vi "Correlation.vi"(6 "zero lag +":i32=1, 7 "Time step (ms)":dbl, 9 "AC final pts":i32, 10 "counts/bin":dbl[](array[numeric]), 11 "mean":dbl) -> (0 "Time":dbl[](array[numeric]), 3 "Data out":dbl[](array[numeric]))   [LabVIEW 2022 SP3]
uses:
  <vilib>/Analysis/2dsp.llb/1D Cross Correlation (DBL).vi
  <vilib>/Analysis/NI_AALPro.lvlib
panel:
  out "Data out 2":dbl[](array[numeric])
  out "elements":dbl[](array[numeric])
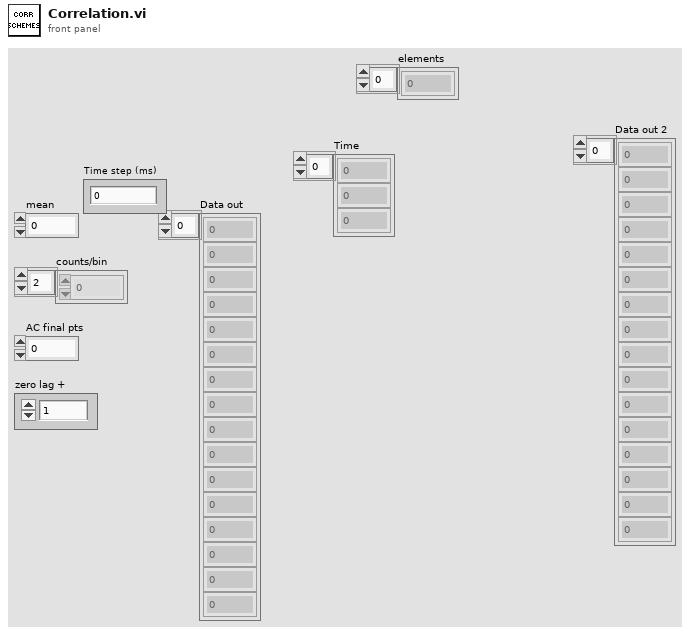
[diagram p1: front panel]
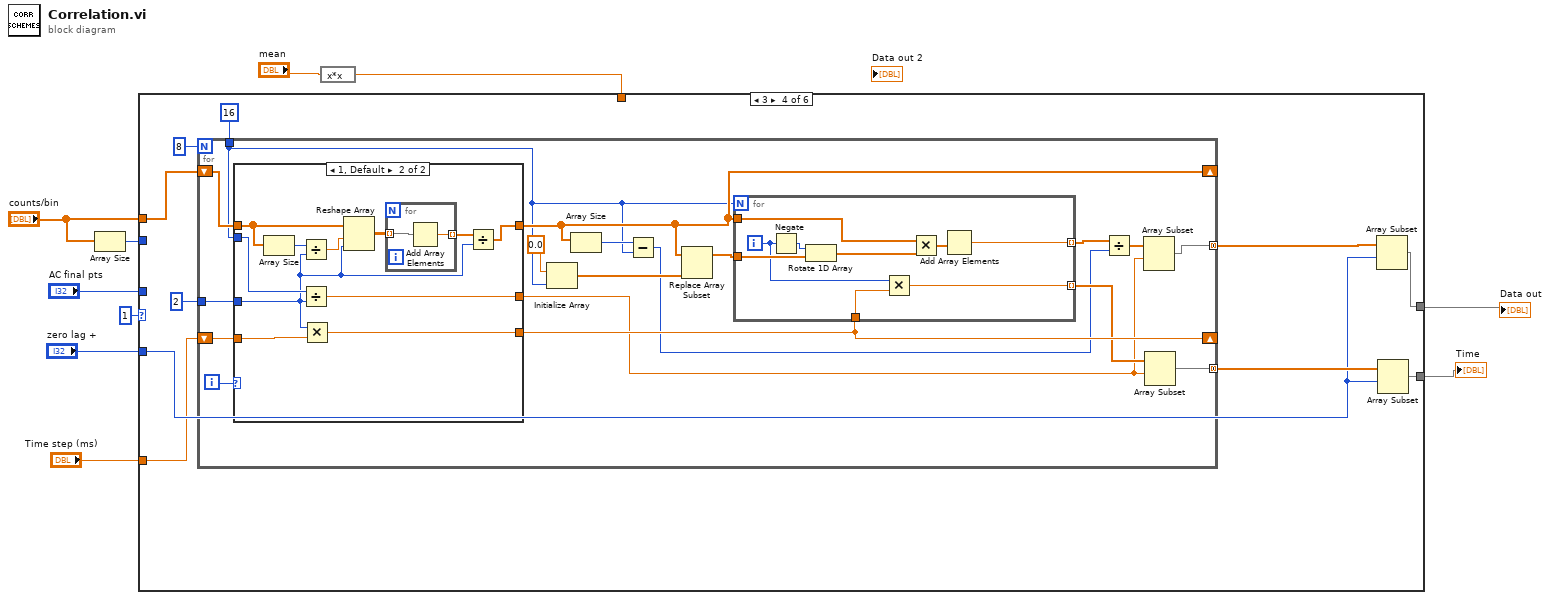
[diagram p0: block diagram]
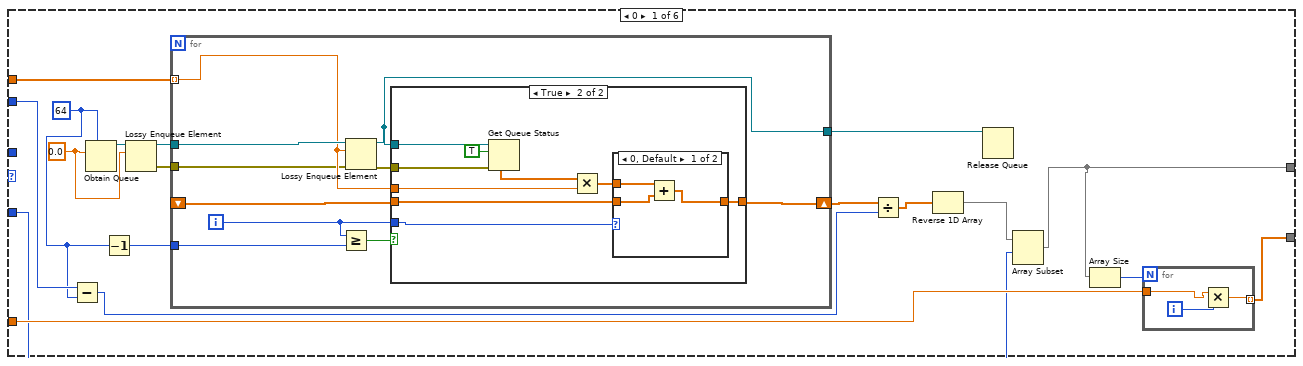
[diagram p2: hidden frame]
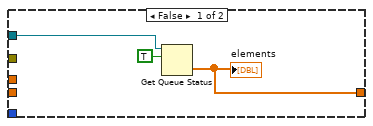
[diagram p3: hidden frame]
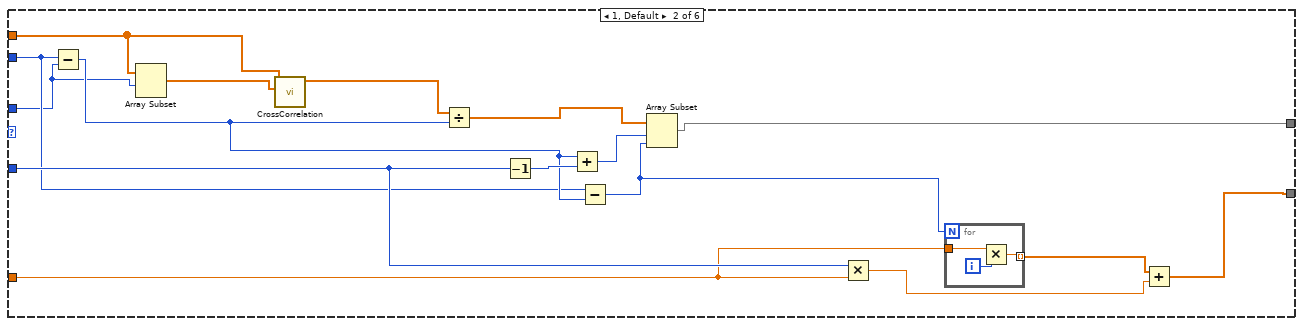
[diagram p5: hidden frame]
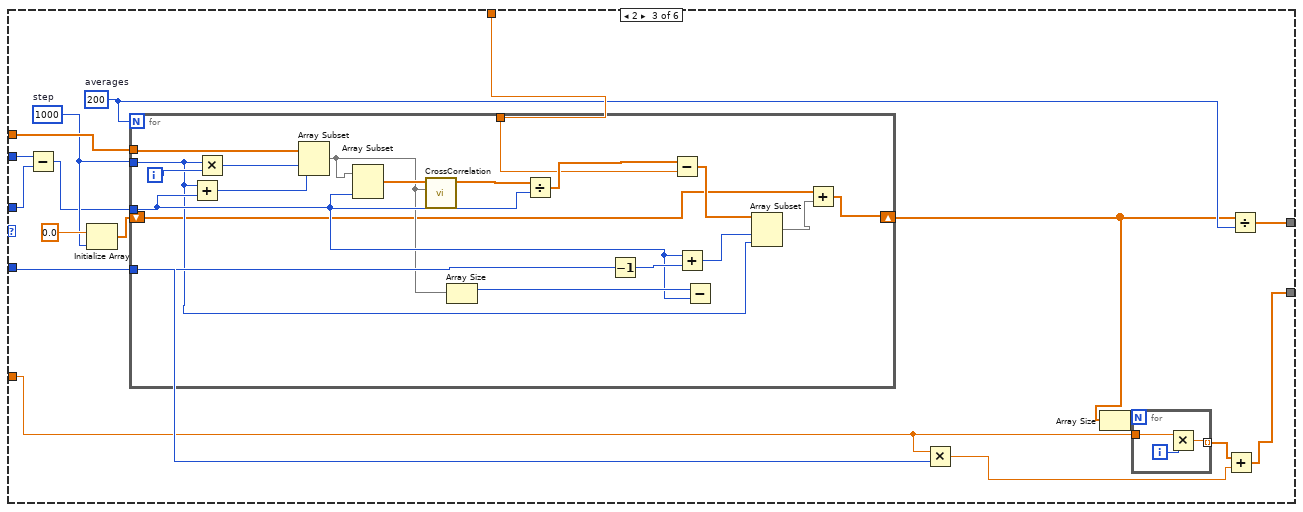
[diagram p6: hidden frame]
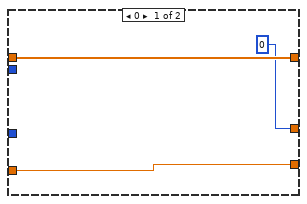
[diagram p7: hidden frame]
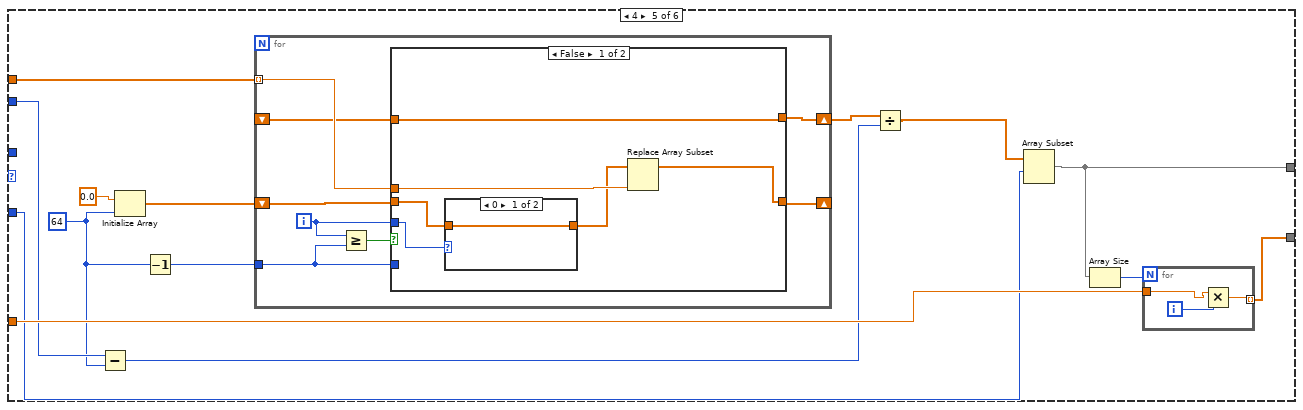
[diagram p8: hidden frame]
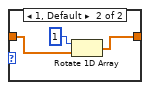
[diagram p9: hidden frame]
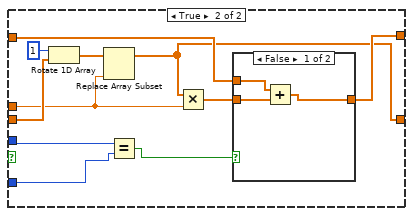
[diagram p10: hidden frame]
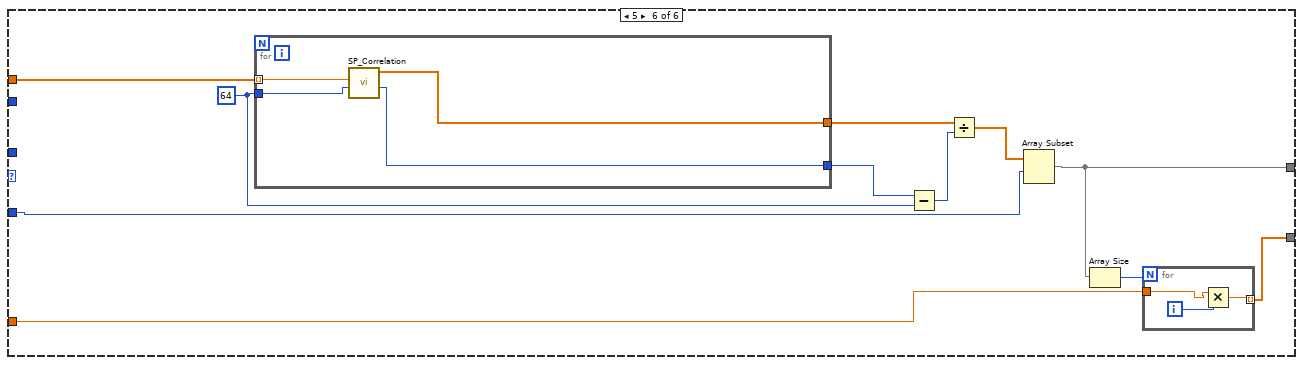
[diagram p12: hidden frame]
diagram:
  n1 = Array Size(array="counts/bin") -> (size(s)=w1:i32)
  n2 = expression code="x*x"("mean") -> (w5:dbl)
  n3 = case shown="3" 1 {
    tunnel: [w17 w58 w90 w121 w170 w223] -> w10
    tunnel: w5 -> [_ _ w93 _ _ _]
    tunnel: "AC final pts" -> [_ w62 w77 _ _ _]
    tunnel: "counts/bin" -> [w28 w60 w92 w125 w182 w229]
    tunnel: "zero lag +" -> [w15 w67 w85 w119 w171 w224]
    tunnel: "Time step (ms)" -> [w25 w66 w84 w118 w180 w227]
    tunnel: [w24 w65 w81 w117 w179 w226] -> w3
    tunnel: w1 -> [w22 w63 w79 _ w175 _]
    frame 0 {
      w11 = 0.0 ("mean")
      w16 = 64 ("max queue size (-1, unlimited)")
      n4 = Subtract(x=w22, y=w16) -> (x-y=w19:i32)
      n5 = Obtain Queue(max queue size (-1, unlimited)=w16, element data type=w11) -> (queue out=w14:refnum<queue>)  [unwired: 3 in, 2 out]
      n6 = Decrement(x=w16) -> (x-1=w23:i32)
      n7 = Lossy Enqueue Element(queue=w14, element=w11) -> (queue out=w13:refnum<queue>, error out=w12:errorcluster)  [unwired: 1 in, 2 out]
      n8 = for {
        tunnel: w28 -> [w37] mode=indexing
        tunnel: w13 -> [w41]
        shift-right: [w39] -> w21
        shift-left: _ -> [w40]
        tunnel: w23 -> [w38]
        tunnel: [w36] -> w27
        tunnel: w12 -> [w32]
        i -> [w33]
        n9 = Greater Or Equal?(x=w33, y=w38) -> (x >= y?=w34:bool)
        n10 = Lossy Enqueue Element(queue=w41, element=w37, error in (no error)=w32) -> (queue out=w36:refnum<queue>, error out=w35:errorcluster)  [unwired: 2 out]
        n11 = case shown="True" w34 {
          tunnel: w36 -> [w43 w53]
          tunnel: w37 -> [_ w45]
          tunnel: w40 -> [_ w52]
          tunnel: [w42 w51] -> w39
          tunnel: w35 -> [_ w50]
          tunnel: w33 -> [_ w47]
          frame False {
            n12 = Get Queue Status(queue=w43, return elements? (F)=TRUE) -> (elements=w42:dbl[])  [unwired: 1 in, 7 out]
            "elements" <- w42
          }
          frame True {
            n13 = Get Queue Status(queue=w53, return elements? (F)=TRUE, error in (no error)=w50) -> (elements=w46:dbl[])  [unwired: 7 out]
            n14 = Multiply(x=w46, y=w45) -> (x*y=w48:dbl[])
            n15 = case shown="0, Default" w47 {
              tunnel: w52 -> [w56 _]
              tunnel: [w54 w57] -> w51
              tunnel: w48 -> [w55 w57]
              frame 0, Default {
                n16 = Add(x=w55, y=w56) -> (x+y=w54:dbl[])
              }
              frame 16 {
              }
            }
          }
        }
      }
      n17 = Divide(x=w21, y=w19) -> (x/y=w20:dbl[])
      n18 = Reverse 1D Array(array=w20) -> (reversed array=w18:dbl[])
      n19 = Release Queue(queue=w27) -> ()  [unwired: 2 in, 3 out]
      n20 = Array Subset(array=w18, index=w15) -> (w17:dbl[])  [unwired: 1 in]
      n21 = Array Size(array=w17) -> (size(s)=w26:i32)
      n22 = for {
        N: w26 -> [_]
        tunnel: [w30] -> w24 mode=indexing
        tunnel: w25 -> [w29]
        i -> [w31]
        n23 = Multiply(x=w29, y=w31) -> (x*y=w30:dbl)
      }
    }
    frame 1, Default {
      n24 = Subtract(x=w63, y=w62) -> (x-y=w64:i32)
      n25 = Array Subset(array=w60, index=w62) -> (w61:dbl[])  [unwired: 1 in]
      n26 = call-poly <vilib>:"CrossCorrelation.vi"("Y"=w61, "X"=w60) -> ("Rxy"=w71:dbl[])  [unwired: 8 in, 1 out]
      n27 = Divide(x=w71, y=w64) -> (x/y=w59:dbl[])
      n28 = Decrement(x=w67) -> (x-1=w73:i32)
      n29 = Add(x=w64, y=w73) -> (x+y=w72:i32)
      n30 = Subtract(x=w63, y=w64) -> (x-y=w68:i32)
      n31 = Array Subset(array=w59, index=w72, length=w68) -> (w58:dbl[])
      n32 = Multiply(x=w67, y=w66) -> (x*y=w70:dbl)
      n33 = for {
        N: w68 -> [_]
        tunnel: [w75] -> w69 mode=indexing
        tunnel: w66 -> [w74]
        i -> [w76]
        n34 = Multiply(x=w74, y=w76) -> (x*y=w75:dbl)
      }
      n35 = Add(x=w69, y=w70) -> (x+y=w65:dbl[])
    }
    frame 2 {
      w80 = 1000  # step
      w91 = 200  # averages
      n36 = Subtract(x=w79, y=w77) -> (x-y=w78:i32)
      n37 = Initialize Array(0.0 ("mean"), w80) -> (w89:dbl[])
      n38 = for {
        N: w91 -> [_]
        tunnel: w78 -> [w103]
        tunnel: w85 -> [w110]
        tunnel: w93 -> [w107]
        tunnel: w92 -> [w106]
        tunnel: w80 -> [w100]
        shift-right: [w98] -> w86
        shift-left: w89 -> [w97]
        i -> [w105]
        n39 = Add(x=w100, y=w103) -> (x+y=w102:i32)
        n40 = Multiply(x=w100, y=w105) -> (x*y=w104:i32)
        n41 = Array Subset(array=w106, index=w104, length=w102) -> (w101:dbl[])
        n42 = Array Subset(array=w101, length=w103) -> (w113:dbl[])  [unwired: 1 in]
        n43 = call-poly <vilib>:"CrossCorrelation.vi"("Y"=w101, "X"=w113) -> ("Rxy"=w112:dbl[])  [unwired: 8 in, 1 out]
        n44 = Array Size(array=w101) -> (size(s)=w111:i32)
        n45 = Divide(x=w112, y=w103) -> (x/y=w109:dbl[])
        n46 = Decrement(x=w110) -> (x-1=w115:i32)
        n47 = Subtract(x=w109, y=w107) -> (x-y=w108:dbl[])
        n48 = Add(x=w103, y=w115) -> (x+y=w114:i32)
        n49 = Subtract(x=w111, y=w103) -> ()  [unwired: 1 out]
        n50 = Array Subset(array=w108, index=w114, length=w100) -> (w99:dbl[])
        n51 = Add(x=w97, y=w99) -> (x+y=w98:dbl[])
      }
      n52 = Multiply(x=w84, y=w85) -> (x*y=w83:dbl)
      n53 = Array Size(array=w86) -> (size(s)=w87:i32)
      n54 = for {
        N: w87 -> [_]
        tunnel: [w95] -> w82 mode=indexing
        tunnel: w84 -> [w94]
        i -> [w96]
        n55 = Multiply(x=w94, y=w96) -> (x*y=w95:dbl)
      }
      n56 = Add(x=w82, y=w83) -> (x+y=w81:dbl[])
      n57 = Divide(x=w86, y=w91) -> (x/y=w90:dbl[])
    }
    frame 3 {
      n58 = for {
        N: 8 -> [_]
        shift-right: [w138] -> _
        shift-left: w125 -> [w139]
        tunnel: 2 -> [w135]
        tunnel: [w128] -> w122 mode=concatenating
        shift-right: [w132] -> _
        shift-left: w118 -> [w133]
        tunnel: [w129] -> w120 mode=concatenating
        tunnel: 16 -> [w126]
        i -> [w134]
        n59 = case shown="1, Default" w134 {
          tunnel: w139 -> [w146 w153]
          tunnel: [w146 w147] -> w138
          tunnel: w135 -> [_ w149]
          tunnel: [0 w150] -> w130
          tunnel: w133 -> [w144 w154]
          tunnel: [w144 w152] -> w132
          tunnel: w126 -> [_ w151]
          frame 0 {
          }
          frame 1, Default {
            n60 = Array Size(array=w153) -> (size(s)=w157:i32)
            n61 = Divide(x=w157, y=w149) -> (x/y=w156:dbl)
            n62 = Divide(x=w151, y=w149) -> (x/y=w150:dbl)
            n63 = Multiply(x=w149, y=w154) -> (x*y=w152:dbl)
            n64 = Reshape Array(w153, w156, w149) -> (w155:dbl[][])
            n65 = for {
              tunnel: w155 -> [w159] mode=indexing
              tunnel: [w158] -> w148 mode=indexing
              n66 = Add Array Elements(numeric array=w159) -> (sum=w158:dbl)
            }
            n67 = Divide(x=w148, y=w149) -> (x/y=w147:dbl[])
          }
        }
        n68 = Initialize Array(0.0 ("mean"), w126) -> (w142:dbl[])
        n69 = Array Size(array=w138) -> (size(s)=w141:i32)
        n70 = Subtract(x=w141, y=w126) -> (x-y=w127:i32)
        n71 = Replace Array Subset(array=w138, new element=w142) -> (w140:dbl[])  [unwired: 1 in]
        n72 = for {
          N: w126 -> [_]
          tunnel: w138 -> [w165]
          tunnel: [w168] -> w137 mode=indexing
          tunnel: w140 -> [w164]
          tunnel: w132 -> [w163]
          tunnel: [w161] -> w131 mode=indexing
          i -> [w162]
          n73 = Negate(x=w162) -> (-x=w160:i32)
          n74 = Rotate 1D Array(1:w164, 2:w160) -> (0:w166:dbl[])
          n75 = Multiply(x=w162, y=w163) -> (x*y=w161:dbl)
          n76 = Multiply(x=w165, y=w166) -> (x*y=w167:dbl[])
          n77 = Add Array Elements(numeric array=w167) -> (sum=w168:dbl)
        }
        n78 = Divide(x=w137, y=w127) -> (x/y=w136:dbl[])
        n79 = Array Subset(array=w136, index=w130) -> (w128:dbl[])  [unwired: 1 in]
        n80 = Array Subset(array=w131, index=w130) -> (w129:dbl[])  [unwired: 1 in]
      }
      n81 = Array Subset(array=w122, index=w119) -> (w121:dbl[])  [unwired: 1 in]
      n82 = Array Subset(array=w120, index=w119) -> (w117:dbl[])  [unwired: 1 in]
    }
    frame 4 {
      w174 = 64 ("max queue size (-1, unlimited)")
      n83 = Subtract(x=w175, y=w174) -> (x-y=w173:i32)
      n84 = Initialize Array(0.0 ("dimension size"), w174) -> (w177:dbl[])
      n85 = Decrement(x=w174) -> (x-1=w176:i32)
      n86 = for {
        tunnel: w182 -> [w191] mode=indexing
        shift-right: [w192] -> _
        shift-left: w177 -> [w193]
        shift-right: [w189] -> w172
        shift-left: _ -> [w188]
        tunnel: w176 -> [w186]
        i -> [w187]
        n87 = Greater Or Equal?(x=w187, y=w186) -> (x >= y?=w190:bool)
        n88 = case shown="False" w190 {
          tunnel: w191 -> [w199 w207]
          tunnel: w193 -> [w197 w214]
          tunnel: [w195 w208] -> w192
          tunnel: [w194 w211] -> w189
          tunnel: w188 -> [w194 w210]
          tunnel: w187 -> [w198 w206]
          tunnel: w186 -> [_ w204]
          frame False {
            n89 = case shown="0" w198 {
              tunnel: w197 -> [w200 w202]
              tunnel: [w200 w201] -> w196
              frame 0 {
              }
              frame 1, Default {
                n90 = Rotate 1D Array(1:w202, 2:1 ("n")) -> (0:w201:dbl[])
              }
            }
            n91 = Replace Array Subset(array=w196, new element=w199) -> (w195:dbl[])  [unwired: 1 in]
          }
          frame True {
            n92 = Rotate 1D Array(1:w214, 2:1 ("n")) -> (0:w212:dbl[])
            n93 = Replace Array Subset(array=w212, new element=w207) -> (w208:dbl[])  [unwired: 1 in]
            n94 = Equal?(x=w206, y=w204) -> (x = y?=w205:bool)
            n95 = Multiply(x=w208, y=w207) -> (x*y=w213:dbl[])
            n96 = case shown="False" w205 {
              tunnel: w213 -> [w217 w218]
              tunnel: [w215 w218] -> w211
              tunnel: w210 -> [w216 _]
              frame False {
                n97 = Add(x=w216, y=w217) -> (x+y=w215:dbl[])
              }
              frame True {
              }
            }
          }
        }
      }
      n98 = Divide(x=w172, y=w173) -> (x/y=w169:dbl[])
      n99 = Array Subset(array=w169, index=w171) -> (w170:dbl[])  [unwired: 1 in]
      n100 = Array Size(array=w170) -> (size(s)=w181:i32)
      n101 = for {
        N: w181 -> [_]
        tunnel: [w184] -> w179 mode=indexing
        tunnel: w180 -> [w183]
        i -> [w185]
        n102 = Multiply(x=w183, y=w185) -> (x*y=w184:dbl)
      }
    }
    frame 5 {
      w221 = 64 ("max queue size (-1, unlimited)")
      n103 = for {
        tunnel: w229 -> [w236] mode=indexing
        tunnel: w221 -> [w235]
        tunnel: [w234] -> w220
        tunnel: [w233] -> w219
        n104 = call "SP_Correlation.vi"("Tau Number"=w235, "New Count"=w236) -> ("interation"=w233:i64, "Cross Corr"=w234:dbl[])  [unwired: 8 in]
      }
      n105 = Subtract(x=w219, y=w221) -> (x-y=w225:i64)
      n106 = Divide(x=w220, y=w225) -> (x/y=w222:dbl[])
      n107 = Array Subset(array=w222, index=w224) -> (w223:dbl[])  [unwired: 1 in]
      n108 = Array Size(array=w223) -> (size(s)=w228:i32)
      n109 = for {
        N: w228 -> [_]
        tunnel: [w231] -> w226 mode=indexing
        tunnel: w227 -> [w230]
        i -> [w232]
        n110 = Multiply(x=w230, y=w232) -> (x*y=w231:dbl)
      }
    }
  }
  "Data out" <- w10
  "Time" <- w3
